vi "CloseBuild.vi"(8 "error in (no error)":errorcluster, 9 "GeneratedFiles":path[](array[path]), 10 "GeneratedDirectories":path[](array[path]), 11 "Build in":refnum<class "AB_Build.lvclass">) -> (0 "error out":errorcluster, 1 "GeneratedFiles out":path[](array[path]), 3 "Build out":refnum<class "AB_Build.lvclass">)   [LabVIEW 2020, in "AB_Build.lvclass"]
uses:
  <vilib>/AppBuilder/AB_Classes/Build/AB_Build.lvclass
  <vilib>/AppBuilder/AB_Classes/Build/AB_Build.lvclass/AB_Build.ctl
  <vilib>/AppBuilder/logging/AB_Log_File_Action.ctl
  <vilib>/AppBuilder/AB_Log_Error_Usage_Data_Type.ctl
  <resource>/Framework/Providers/Common/provcom_StringGlobals.vi
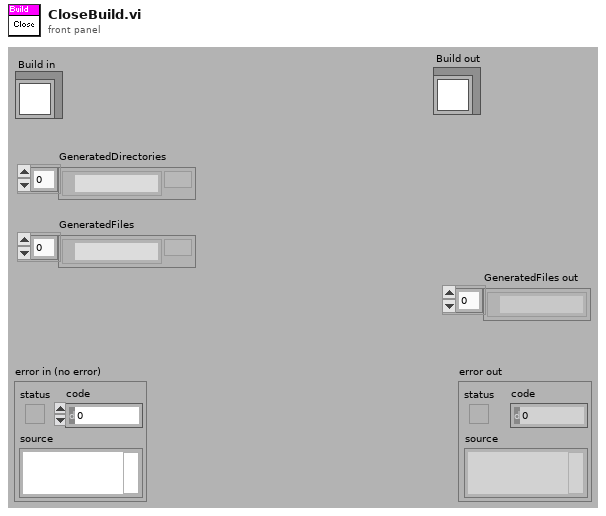
[diagram p1: front panel]
types:
  T1 = typedef "AB_Log_File_Action.ctl" = enum16{"write", "open", "close"}
  T2 = typedef "AB_Log_Error_Usage_Data_Type.ctl" = enum16{"NI_APP_BUILDER_ERROR", "NI_INSTALLER_BUILDER_ERROR"}
  T3 = typedef "provcom_ProgressBar_Events.ctl" = cluster{"newJob":refnum<user-event>, "newItem":refnum<user-event>, "errorMsg":T4, "cancel":refnum<user-event>}
  T4 = typedef "mxLvBuildError.ctl" = refnum<user-event>
  T5 = cluster{"major":u16, "minor":u16, "patch":u16, "build":u16}
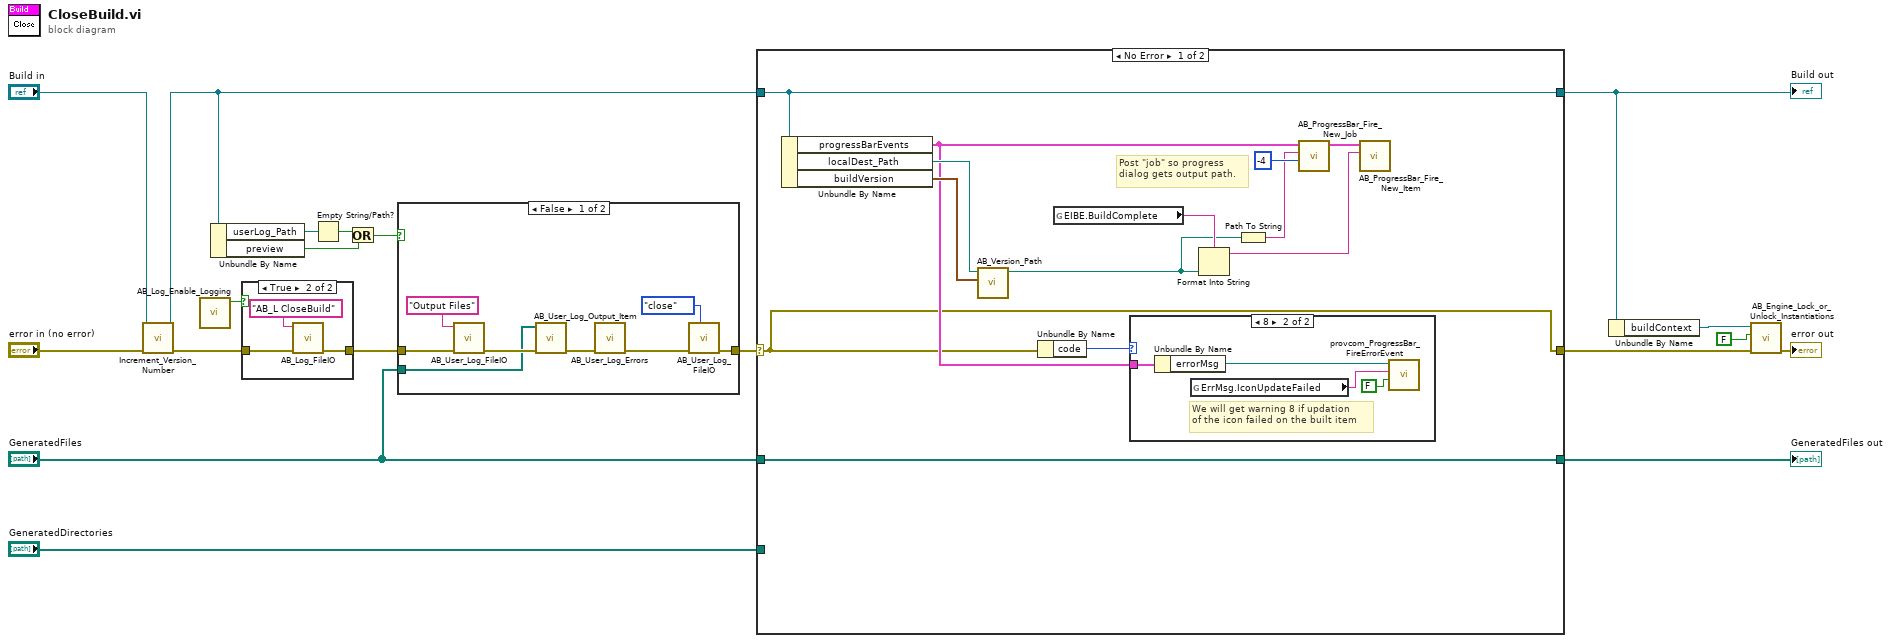
[diagram p0: block diagram]
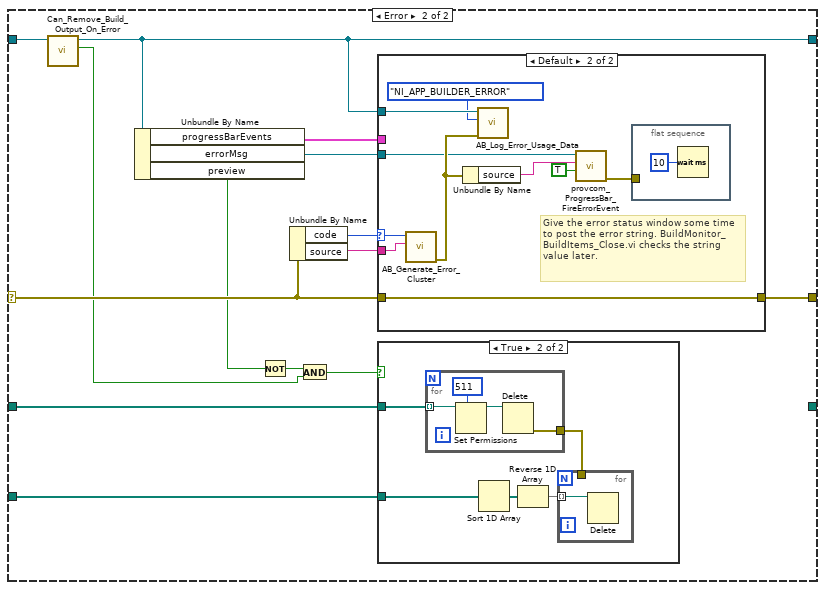
[diagram p5: hidden frame]
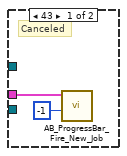
[diagram p7: hidden frame]
diagram:
  n1 = call-dynamic "Increment_Version_Number.vi"("error in (no error)"="error in (no error)", "AB_Build in"="Build in") -> ("error out"=w3:errorcluster, "AB_Build out"=w1:refnum<class "AB_Build.lvclass">)  [unwired: 1 in, 7 out]
  n2 = call <vilib>:"AB_Log_Enable_Logging.vi"() -> ("log?"=w13:bool)  [unwired: 2 in, 9 out]
  n3 = Unbundle By Name(w1) -> ("userLog_Path"=w17:path, "preview"=w6:bool)
  n4 = case shown="True" w13 {
    tunnel: w3 -> [w20 w23]
    tunnel: [w20 w22] -> w14
    frame False {
    }
    frame True {
      n5 = call <vilib>:"AB_Log_FileIO.vi"("error in (no error)"=w23, "newSection"="AB_L CloseBuild" ("sectionName")) -> ("error out"=w22:errorcluster)  [unwired: 3 in, 6 out]
    }
  }
  n6 = Empty String/Path?(string/path=w17) -> (empty?=w7:bool)
  n7 = Or(x=w7, y=w6) -> (x .or. y?=w5:bool)
  n8 = case shown="False" w5 {
    tunnel: w14 -> [w28 w32]
    tunnel: [w31 w32] -> w16
    tunnel: "GeneratedFiles" -> [w26 _]
    frame False {
      n9 = call <vilib>:"AB_User_Log_FileIO.vi"("error in (no error)"=w28, "newSection"="Output Files") -> ("error out"=w27:errorcluster)  [unwired: 3 in, 6 out]
      n10 = call <vilib>:"AB_User_Log_Output_Item.vi"("error in (no error)"=w27, "outputFilePaths"=w26) -> ("error out"=w25:errorcluster)  [unwired: 9 out]
      n11 = call <vilib>:"AB_User_Log_Errors.vi"("error in (no error)"=w25) -> ("error out"=w24:errorcluster)  [unwired: 10 out]
      n12 = call <vilib>:"AB_User_Log_FileIO.vi"("fileAction"=AB_Log_File_Action."close", "error in (no error)"=w24) -> ("error out"=w31:errorcluster)  [unwired: 3 in, 6 out]
    }
    frame True {
    }
  }
  n13 = case shown="No Error" w16 {
    selector: w16 -> [w33 w60]
    tunnel: [w33 w61] -> w9
    tunnel: [w36 w50] -> w10
    tunnel: w1 -> [w36 w54]
    tunnel: "GeneratedFiles" -> [w44 w58]
    tunnel: [w44 _] -> w19
    tunnel: "GeneratedDirectories" -> [_ w57]
    frame No Error {
      # "Post \"job\" so progress dialog gets output path."
      n14 = Unbundle By Name(w36) -> ("progressBarEvents"=w34:T3, "localDest_Path"=w39:path, "buildVersion"=w38:T5)
      n15 = call <vilib>:"AB_Version_Path.vi"("buildVersion"=w38, "unversioned path"=w39) -> ("versioned path"=w37:path)  [unwired: 9 in]
      n16 = Unbundle By Name(w33) -> ("code"=w35:i32)
      n17 = global read "provcom_StringGlobals.vi" "EIBE.BuildComplete"() -> (w45:string)
      n18 = case shown="8" w35 {
        tunnel: w34 -> [_ w48]
        frame Default {
        }
        frame 8 {
          # "We will get warning 8 if updation \nof the icon failed on the built item"
          n19 = Unbundle By Name(w48) -> ("errorMsg"=w49:T4)
          n20 = global read "provcom_StringGlobals.vi" "ErrMsg.IconUpdateFailed"() -> (w46:string)
          n21 = call <resource>:"provcom_ProgressBar_FireErrorEvent.vi"("Error?"=FALSE, "ErrorText"=w46, "Error event"=w49) -> ()  [unwired: 8 in, 1 out]
        }
      }
      n22 = Format Into String(format string=w45, w37) -> (resulting string=w42:string)  [unwired: 2 in, 1 out]
      n23 = Path To String(path=w37) -> (string=w40:string)
      n24 = call <vilib>:"AB_ProgressBar_Fire_New_Job.vi"("#ofItems"=-4, "Label"=w40, "progressBarEvents in"=w34) -> ("progressBarEvents out"=w41:T3)  [unwired: 1 in, 7 out]
      n25 = call <vilib>:"AB_ProgressBar_Fire_New_Item.vi"("Label"=w42, "progressBarEvents in"=w41) -> ()  [unwired: 1 in, 9 out]
    }
    frame Error {
      n26 = call-dynamic "Can_Remove_Build_Output_On_Error.vi"("Build in"=w54) -> ("Remove build output"=w51:bool, "Build out"=w50:refnum<class "AB_Build.lvclass">)  [unwired: 8 in, 1 out]
      n27 = Unbundle By Name(w50) -> ("progressBarEvents"=w59:T3, "errorMsg"=w56:T4, "preview"=w55:bool)
      n28 = Not(x=w55) -> (.not. x?=w53:bool)
      n29 = Unbundle By Name(w60) -> ("code"=w62:i32, "source"=w63:string)
      n30 = And(x=w53, y=w51) -> (x .and. y?=w52:bool)
      n31 = case shown="Default" w62 {
        selector: w62 -> [_ w84]
        tunnel: w63 -> [_ w83]
        tunnel: [_ w85] -> w61
        tunnel: w60 -> [_ w85]
        tunnel: w59 -> [w74 _]
        tunnel: w56 -> [_ w79]
        tunnel: w50 -> [_ w81]
        frame 43 {
          # "Canceled"
          n32 = call <vilib>:"AB_ProgressBar_Fire_New_Job.vi"("#ofItems"=-1, "progressBarEvents in"=w74) -> ()  [unwired: 2 in, 8 out]
        }
        frame Default {
          # "Give the error status window some time to post the error string. BuildMonitor_BuildItems_Close.vi checks the string value later."
          n33 = call <vilib>:"AB_Generate_Error_Cluster.vi"("source"=w83, "Code"=w84) -> ("error out"=w82:errorcluster)  [unwired: 9 in]
          n34 = Unbundle By Name(w82) -> ("source"=w78:string)
          n35 = call <vilib>:"AB_Log_Error_Usage_Data.vi"("Error In"=w82, "CEIP Key (NI_APP_BUILDER_ERROR)"=AB_Log_Error_Usage_Data_Type."NI_APP_BUILDER_ERROR", "Build class"=w81) -> ()  [unwired: 8 in, 1 out]
          n36 = call <resource>:"provcom_ProgressBar_FireErrorEvent.vi"("Error?"=TRUE, "ErrorText"=w78, "Error event"=w79) -> ("error out"=w77:errorcluster)  [unwired: 8 in]
          n37 = flat-sequence {
            tunnel: w77 -> [_]
            frame #0 {
              n38 = Wait (ms)(milliseconds to wait=u32 10) -> ()  [unwired: 1 out]
            }
          }
        }
      }
      n39 = case shown="True" w52 {
        tunnel: w58 -> [_ w68]
        tunnel: w57 -> [_ w67]
        frame False {
        }
        frame True {
          n40 = for {
            tunnel: [w70] -> w64
            tunnel: w68 -> [w69] mode=indexing
            n41 = Set Permissions(7:i16 511 ("permissions"), 11:w69) -> (3:w72:path)  [unwired: 1 in, 3 out]
            n42 = Delete(path (use dialog)=w72) -> (error out=w70:errorcluster)  [unwired: 1 in, 5 out]
          }
          n43 = Sort 1D Array(array=w67) -> (sorted array=w65:path[])
          n44 = Reverse 1D Array(array=w65) -> (reversed array=w66:path[])
          n45 = for {
            tunnel: w66 -> [w73] mode=indexing
            tunnel: w64 -> [_]
            n46 = Delete(path (use dialog)=w73) -> ()  [unwired: 1 in, 6 out]
          }
        }
      }
    }
  }
  "GeneratedFiles out" <- w19
  "Build out" <- w10
  n47 = Unbundle By Name(w10) -> ("buildContext"=w12:refnum<vi>)
  n48 = call <vilib>:"AB_Engine_Lock_or_Unlock_Instantiations.vi"("error in"=w9, "Lock?"=FALSE, "Instance to Lock or Unlock"=w12) -> ("error out"=→"error out":errorcluster)  [unwired: 8 in]
